vi "tale of three indices - integer.vi"(4 "right most":i32, 6 "left most":i32, 7 "selector":T1(ring), 8 "window":i32, 9 "right":i32, 10 "center":i32, 11 "left":i32) -> (0 "window out":i32, 1 "right out":i32, 2 "center out":i32, 3 "left out":i32, 5 "selector out":T1(ring))   [LabVIEW 2010]
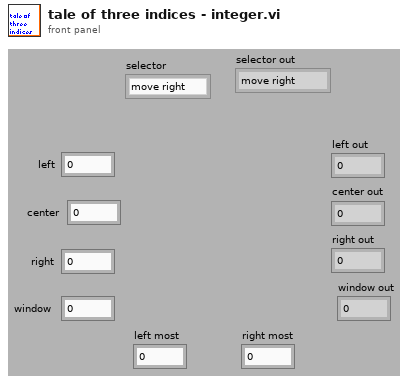
[diagram p1: front panel]
types:
  T1 = enum16{"move right", "move left", "balance", "shrink", "broaden", "do nothing", "reset", "check"}
  T2 = enum16{"not a number", "above", "in range", "below"}
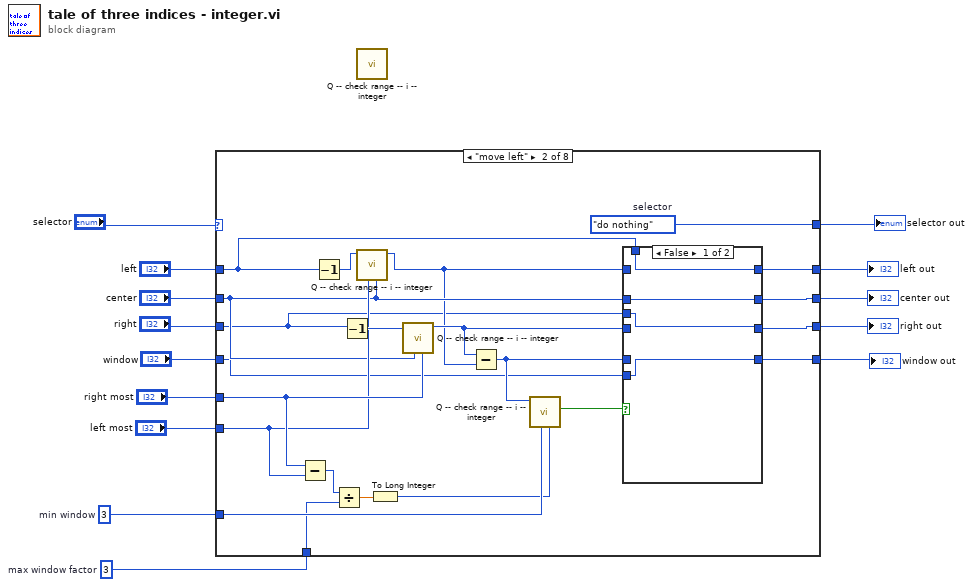
[diagram p0: block diagram]
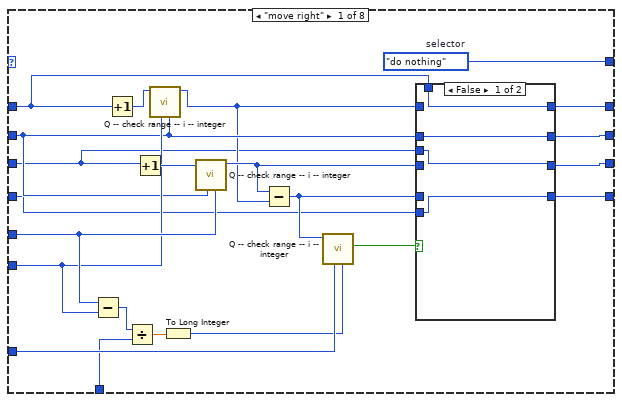
[diagram p2: hidden frame]
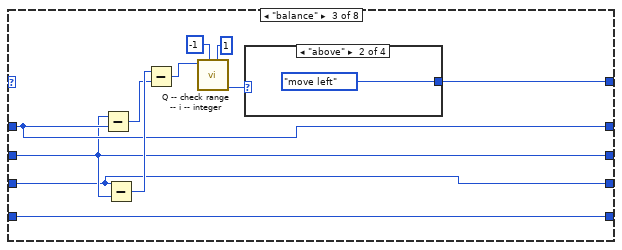
[diagram p5: hidden frame]
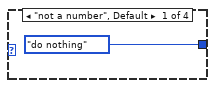
[diagram p6: hidden frame]
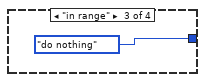
[diagram p7: hidden frame]
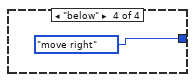
[diagram p8: hidden frame]
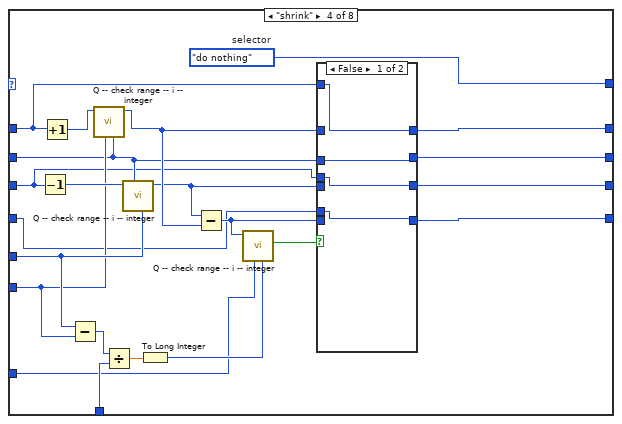
[diagram p9: hidden frame]
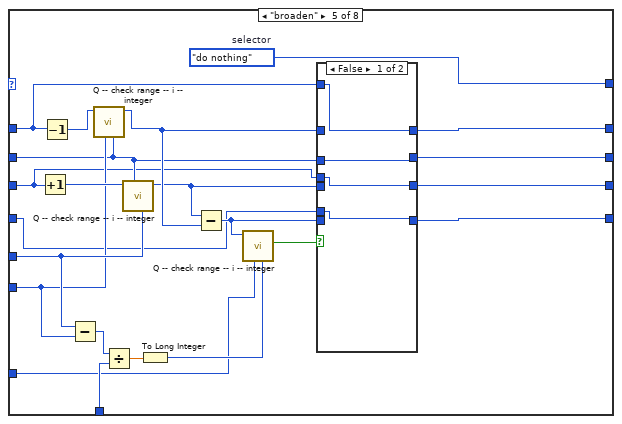
[diagram p11: hidden frame]
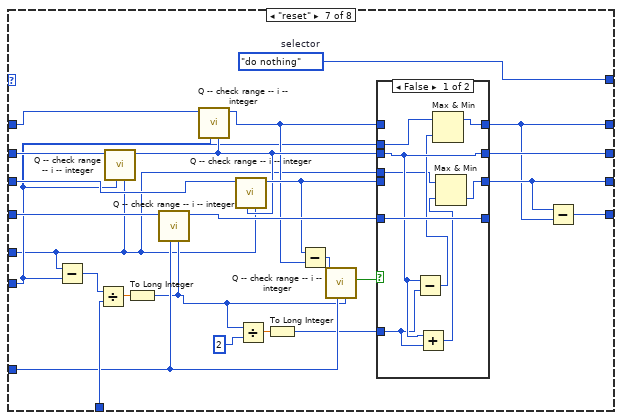
[diagram p14: hidden frame]
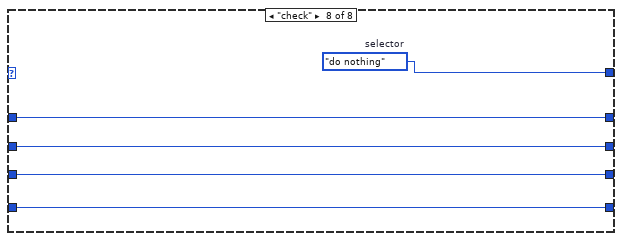
[diagram p16: hidden frame]
diagram:
  w2 = 3  # max window factor
  w1 = 3  # min window
  n1 = case shown="\"move left\"" "selector" {
    selector: "selector" -> [_ _ _ _ _ w153 _ _]
    tunnel: "left" -> [w16 w46 w77 w93 w123 w154 w174 w197]
    tunnel: [w21 w51 w76 w99 w129 w152 w167 w196] -> w13
    tunnel: "center" -> [w20 w50 w76 w98 w128 w152 w175 w196]
    tunnel: [w19 w49 w77 w101 w131 w154 w155 w197] -> w11
    tunnel: "right" -> [w15 w45 w75 w92 w122 w151 w173 w195]
    tunnel: "right most" -> [w30 w60 _ w109 w139 _ w158 _]
    tunnel: [w23 w53 w75 w97 w127 w151 w156 w195] -> w8
    tunnel: [w25 w55 w78 w95 w125 w150 w157 w194] -> w7
    tunnel: "window" -> [w17 w47 w78 w91 w121 w150 w179 w194]
    tunnel: "left most" -> [w29 w59 _ w108 w138 _ w159 _]
    tunnel: [w34 w64 w79 w90 w120 w153 w164 w193] -> w4
    tunnel: w2 -> [w28 w58 _ w106 w136 _ w177 _]
    tunnel: w1 -> [w33 w63 _ w103 w133 _ w171 _]
    frame "move right" {
      w34 = T1."do nothing"  # selector
      n2 = Subtract(x=w30, y=w29) -> (x-y=w32:i32)
      n3 = Increment(x=w16) -> (x+1=w36:i32)
      n4 = Divide(x=w32, y=w28) -> (x/y=w31:dbl)
      n5 = Increment(x=w15) -> (x+1=w35:i32)
      n6 = call "Q -- check range -- i -- integer.vi"("upper"=w20, "lower"=w29, "number"=w36) -> ("number in range"=w18:i32)  [unwired: 6 in, 2 out]
      n7 = To Long Integer(number=w31) -> (32bit integer=w27:i32)
      n8 = call "Q -- check range -- i -- integer.vi"("upper"=w30, "lower"=w20, "number"=w35) -> ("number in range"=w22:i32)  [unwired: 6 in, 2 out]
      n9 = Subtract(x=w22, y=w18) -> (x-y=w24:i32)
      n10 = call "Q -- check range -- i -- integer.vi"("upper"=w27, "lower"=w33, "number"=w24) -> ("in range?"=w26:bool)  [unwired: 6 in, 2 out]
      n11 = case shown="False" w26 {
        tunnel: [w39 w44] -> w25
        tunnel: w24 -> [_ w44]
        tunnel: [w37 w43] -> w23
        tunnel: w22 -> [_ w43]
        tunnel: [w40 w42] -> w21
        tunnel: w20 -> [w40 w42]
        tunnel: [w38 w41] -> w19
        tunnel: w18 -> [_ w41]
        tunnel: w17 -> [w39 _]
        tunnel: w16 -> [w38 _]
        tunnel: w15 -> [w37 _]
        frame False {
        }
        frame True {
        }
      }
    }
    frame "move left" {
      w64 = T1."do nothing"  # selector
      n12 = Subtract(x=w60, y=w59) -> (x-y=w62:i32)
      n13 = Decrement(x=w46) -> (x-1=w66:i32)
      n14 = Divide(x=w62, y=w58) -> (x/y=w61:dbl)
      n15 = Decrement(x=w45) -> (x-1=w65:i32)
      n16 = call "Q -- check range -- i -- integer.vi"("upper"=w50, "lower"=w59, "number"=w66) -> ("number in range"=w48:i32)  [unwired: 6 in, 2 out]
      n17 = To Long Integer(number=w61) -> (32bit integer=w57:i32)
      n18 = call "Q -- check range -- i -- integer.vi"("upper"=w60, "lower"=w50, "number"=w65) -> ("number in range"=w52:i32)  [unwired: 6 in, 2 out]
      n19 = Subtract(x=w52, y=w48) -> (x-y=w54:i32)
      n20 = call "Q -- check range -- i -- integer.vi"("upper"=w57, "lower"=w63, "number"=w54) -> ("in range?"=w56:bool)  [unwired: 6 in, 2 out]
      n21 = case shown="False" w56 {
        tunnel: [w69 w74] -> w55
        tunnel: w54 -> [_ w74]
        tunnel: [w67 w73] -> w53
        tunnel: w52 -> [_ w73]
        tunnel: [w70 w72] -> w51
        tunnel: w50 -> [w70 w72]
        tunnel: [w68 w71] -> w49
        tunnel: w48 -> [_ w71]
        tunnel: w47 -> [w69 _]
        tunnel: w46 -> [w68 _]
        tunnel: w45 -> [w67 _]
        frame False {
        }
        frame True {
        }
      }
    }
    frame "balance" {
      n22 = Subtract(x=w76, y=w77) -> (x-y=w84:i32)
      n23 = Subtract(x=w75, y=w76) -> (x-y=w85:i32)
      n24 = Subtract(x=w85, y=w84) -> (x-y=w83:i32)
      n25 = call "Q -- check range -- i -- integer.vi"("upper"=1, "lower"=-1, "number"=w83) -> ("selector"=w80:T2)  [unwired: 6 in, 2 out]
      n26 = case shown="\"above\"" w80 {
        tunnel: [T1."do nothing" ("selector") T1."move left" ("selector") T1."do nothing" ("selector") T1."move right" ("selector")] -> w79
        frame "not a number", Default {
        }
        frame "above" {
        }
        frame "in range" {
        }
        frame "below" {
        }
      }
    }
    frame "shrink" {
      w90 = T1."do nothing"  # selector
      n27 = Decrement(x=w92) -> (x-1=w110:i32)
      n28 = Increment(x=w93) -> (x+1=w111:i32)
      n29 = Subtract(x=w109, y=w108) -> (x-y=w107:i32)
      n30 = call "Q -- check range -- i -- integer.vi"("upper"=w98, "lower"=w108, "number"=w111) -> ("number in range"=w100:i32)  [unwired: 6 in, 2 out]
      n31 = Divide(x=w107, y=w106) -> (x/y=w105:dbl)
      n32 = call "Q -- check range -- i -- integer.vi"("upper"=w109, "lower"=w98, "number"=w110) -> ("number in range"=w96:i32)  [unwired: 6 in, 2 out]
      n33 = To Long Integer(number=w105) -> (32bit integer=w104:i32)
      n34 = Subtract(x=w96, y=w100) -> (x-y=w94:i32)
      n35 = call "Q -- check range -- i -- integer.vi"("upper"=w104, "lower"=w103, "number"=w94) -> ("in range?"=w102:bool)  [unwired: 6 in, 2 out]
      n36 = case shown="False" w102 {
        tunnel: [w115 w119] -> w101
        tunnel: w100 -> [_ w119]
        tunnel: [w114 w118] -> w99
        tunnel: w98 -> [w114 w118]
        tunnel: [w113 w117] -> w97
        tunnel: w96 -> [_ w117]
        tunnel: [w112 w116] -> w95
        tunnel: w94 -> [_ w116]
        tunnel: w93 -> [w115 _]
        tunnel: w92 -> [w113 _]
        tunnel: w91 -> [w112 _]
        frame False {
        }
        frame True {
        }
      }
    }
    frame "broaden" {
      w120 = T1."do nothing"  # selector
      n37 = Increment(x=w122) -> (x+1=w140:i32)
      n38 = Decrement(x=w123) -> (x-1=w141:i32)
      n39 = Subtract(x=w139, y=w138) -> (x-y=w137:i32)
      n40 = call "Q -- check range -- i -- integer.vi"("upper"=w128, "lower"=w138, "number"=w141) -> ("number in range"=w130:i32)  [unwired: 6 in, 2 out]
      n41 = Divide(x=w137, y=w136) -> (x/y=w135:dbl)
      n42 = call "Q -- check range -- i -- integer.vi"("upper"=w139, "lower"=w128, "number"=w140) -> ("number in range"=w126:i32)  [unwired: 6 in, 2 out]
      n43 = To Long Integer(number=w135) -> (32bit integer=w134:i32)
      n44 = Subtract(x=w126, y=w130) -> (x-y=w124:i32)
      n45 = call "Q -- check range -- i -- integer.vi"("upper"=w134, "lower"=w133, "number"=w124) -> ("in range?"=w132:bool)  [unwired: 6 in, 2 out]
      n46 = case shown="False" w132 {
        tunnel: [w145 w149] -> w131
        tunnel: w130 -> [_ w149]
        tunnel: [w144 w148] -> w129
        tunnel: w128 -> [w144 w148]
        tunnel: [w143 w147] -> w127
        tunnel: w126 -> [_ w147]
        tunnel: [w142 w146] -> w125
        tunnel: w124 -> [_ w146]
        tunnel: w123 -> [w145 _]
        tunnel: w122 -> [w143 _]
        tunnel: w121 -> [w142 _]
        frame False {
        }
        frame True {
        }
      }
    }
    frame "do nothing", Default {
    }
    frame "reset" {
      w164 = T1."do nothing"  # selector
      n47 = Subtract(x=w158, y=w159) -> (x-y=w178:i32)
      n48 = Divide(x=w178, y=w177) -> (x/y=w176:dbl)
      n49 = call "Q -- check range -- i -- integer.vi"("upper"=w158, "lower"=w159, "number"=w175) -> ("number in range"=w166:i32)  [unwired: 6 in, 2 out]
      n50 = To Long Integer(number=w176) -> (32bit integer=w162:i32)
      n51 = call "Q -- check range -- i -- integer.vi"("upper"=w162, "lower"=w171, "number"=w179) -> ("number in range"=w169:i32)  [unwired: 6 in, 2 out]
      n52 = call "Q -- check range -- i -- integer.vi"("upper"=w166, "lower"=w159, "number"=w174) -> ("number in range"=w165:i32)  [unwired: 6 in, 2 out]
      n53 = call "Q -- check range -- i -- integer.vi"("upper"=w158, "lower"=w166, "number"=w173) -> ("number in range"=w168:i32)  [unwired: 6 in, 2 out]
      n54 = Divide(x=w162, y=2) -> (x/y=w163:dbl)
      n55 = To Long Integer(number=w163) -> (32bit integer=w160:i32)
      n56 = Subtract(x=w168, y=w165) -> (x-y=w172:i32)
      n57 = call "Q -- check range -- i -- integer.vi"("upper"=w162, "lower"=w171, "number"=w172) -> ("in range?"=w170:bool)  [unwired: 6 in, 2 out]
      n58 = case shown="False" w170 {
        tunnel: [w188 w192] -> _
        tunnel: w169 -> [w188 w192]
        tunnel: [w180 w191] -> w156
        tunnel: w168 -> [_ w191]
        tunnel: [w187 w190] -> w167
        tunnel: w166 -> [w187 w190]
        tunnel: [w183 w189] -> w155
        tunnel: w165 -> [_ w189]
        tunnel: w160 -> [w186 _]
        tunnel: w159 -> [w184 _]
        tunnel: w158 -> [w181 _]
        frame False {
          n59 = Subtract(x=w187, y=w186) -> (x-y=w185:i32)
          n60 = Add(x=w187, y=w186) -> (x+y=w182:i32)
          n61 = Max & Min(x=w184, y=w185) -> (max(x,y)=w183:i32)  [unwired: 1 out]
          n62 = Max & Min(x=w181, y=w182) -> (min(x,y)=w180:i32)  [unwired: 1 out]
        }
        frame True {
        }
      }
      n63 = Subtract(x=w156, y=w155) -> (x-y=w157:i32)
    }
    frame "check" {
      w193 = T1."do nothing"  # selector
    }
  }
  "left out" <- w11
  "center out" <- w13
  "right out" <- w8
  "window out" <- w7
  "selector out" <- w4
  n64 = call "Q -- check range -- i -- integer.vi"() -> ()  [unwired: 9 in, 3 out]
